vi "_Read Tx FIFO.vi"(8 "error in (no error)":errorcluster, 9 "Number of elements":u32, 10 "Channel Number":u32, 11 "Refnum in":T1) -> (0 "error out":errorcluster, 1 "Elements Remaining":u32, 2 "Data":u32[](array[numeric]), 3 "Refnum out":T1)   [LabVIEW 2020, in "985x Support Addon Engine.lvlib"]
uses:
  985x Support Addon Engine.lvlib
  Types/FPGA Refnum.ctl
  <vilib>/Utility/error.llb/Error Cluster From Error Code.vi
  <vilib>/rvi/errors/niLvFpgaAdjustHostInterfaceError.vi
  <vilib>/rvi/interface/nirviMethod/nirviMethod.xnode
  <vilib>/FPGAPlugInAG/Dynamic/niLvFpga_ReadFifo_Dynamic.vi
  <vilib>/rvi/errors/niLvFpgaMergeErrorWithErrorCode.vi
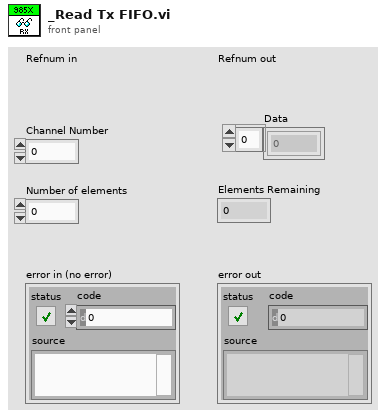
[diagram p1: front panel]
types:
  T1 = typedef "985x Support Addon Engine.lvlib/FPGA Refnum.ctl" = refnum<k20>
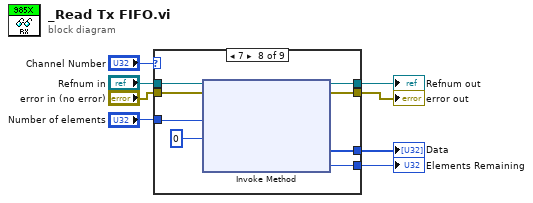
[diagram p0: block diagram]
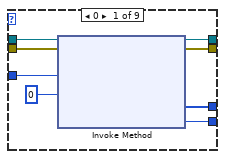
[diagram p2: hidden frame]
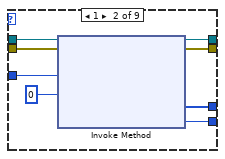
[diagram p3: hidden frame]
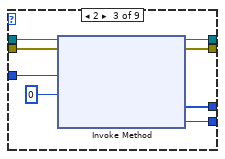
[diagram p4: hidden frame]
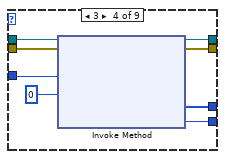
[diagram p5: hidden frame]
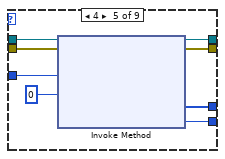
[diagram p6: hidden frame]
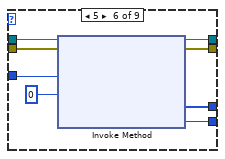
[diagram p7: hidden frame]
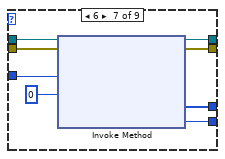
[diagram p8: hidden frame]
diagram:
  n1 = case shown="7" "Channel Number" {
    tunnel: "Refnum in" -> [w16 w24 w32 w40 w48 w56 w64 w72 w74]
    tunnel: "error in (no error)" -> [w15 w23 w31 w39 w47 w55 w63 w71 w73]
    tunnel: [w13 w21 w29 w37 w45 w53 w61 w69 w74] -> w5
    tunnel: [w12 w20 w28 w36 w44 w52 w60 w68 w73] -> w6
    tunnel: [w11 w19 w27 w35 w43 w51 w59 w67 _] -> w7
    tunnel: [w9 w17 w26 w33 w41 w49 w57 w65 _] -> w2
    tunnel: "Number of elements" -> [w10 w18 w25 w34 w42 w50 w58 w66 _]
    frame 0 {
      n2 = xnode "Invoke Method"("FPGA VI Reference In"=w16, "error in"=w15, "Number of Elements"=w10, "Timeout (ms)"=0) -> ("FPGA VI Reference Out"=w13:T1, "error out"=w12:errorcluster, "Data"=w9:u32[], "Elements Remaining"=w11:u32)
    }
    frame 1 {
      n3 = xnode "Invoke Method"("FPGA VI Reference In"=w24, "error in"=w23, "Number of Elements"=w18, "Timeout (ms)"=0) -> ("FPGA VI Reference Out"=w21:T1, "error out"=w20:errorcluster, "Data"=w17:u32[], "Elements Remaining"=w19:u32)
    }
    frame 2 {
      n4 = xnode "Invoke Method"("FPGA VI Reference In"=w32, "error in"=w31, "Number of Elements"=w25, "Timeout (ms)"=0) -> ("FPGA VI Reference Out"=w29:T1, "error out"=w28:errorcluster, "Data"=w26:u32[], "Elements Remaining"=w27:u32)
    }
    frame 3 {
      n5 = xnode "Invoke Method"("FPGA VI Reference In"=w40, "error in"=w39, "Number of Elements"=w34, "Timeout (ms)"=0) -> ("FPGA VI Reference Out"=w37:T1, "error out"=w36:errorcluster, "Data"=w33:u32[], "Elements Remaining"=w35:u32)
    }
    frame 4 {
      n6 = xnode "Invoke Method"("FPGA VI Reference In"=w48, "error in"=w47, "Number of Elements"=w42, "Timeout (ms)"=0) -> ("FPGA VI Reference Out"=w45:T1, "error out"=w44:errorcluster, "Data"=w41:u32[], "Elements Remaining"=w43:u32)
    }
    frame 5 {
      n7 = xnode "Invoke Method"("FPGA VI Reference In"=w56, "error in"=w55, "Number of Elements"=w50, "Timeout (ms)"=0) -> ("FPGA VI Reference Out"=w53:T1, "error out"=w52:errorcluster, "Data"=w49:u32[], "Elements Remaining"=w51:u32)
    }
    frame 6 {
      n8 = xnode "Invoke Method"("FPGA VI Reference In"=w64, "error in"=w63, "Number of Elements"=w58, "Timeout (ms)"=0) -> ("FPGA VI Reference Out"=w61:T1, "error out"=w60:errorcluster, "Data"=w57:u32[], "Elements Remaining"=w59:u32)
    }
    frame 7 {
      n9 = xnode "Invoke Method"("FPGA VI Reference In"=w72, "error in"=w71, "Number of Elements"=w66, "Timeout (ms)"=0) -> ("FPGA VI Reference Out"=w69:T1, "error out"=w68:errorcluster, "Data"=w65:u32[], "Elements Remaining"=w67:u32)
    }
    frame Default {
    }
  }
  "Elements Remaining" <- w7
  "error out" <- w6
  "Refnum out" <- w5
  "Data" <- w2
